vi "Set Digital State.vi"(8 "error in (no error)":errorcluster, 9 "Digital Control State (1: High)":i32(ring)=1 items=["Low", "High"], 10 "Line Number (1: line1)":i32(ring)=1 items=["line1"=1, "line2"=2, "line3"=3, "line4"=4, "line5"=5, "line6"=6], 11 "VISA resource name":refnum<visa-resource-name>) -> (0 "error out":errorcluster, 3 "VISA resource name out":refnum<visa-resource-name>)   [LabVIEW 2023, in "Keithley DMM6500 DAQ6500 Series.lvlib"]
doc: "Sets a digital I/O line high or low when the line is set for digital control and returns the state on the digital I/O lines."
uses:
  <instrlib>/Keithley DMM6500 DAQ6500 Series/Keithley DMM6500 DAQ6500 Series.lvlib
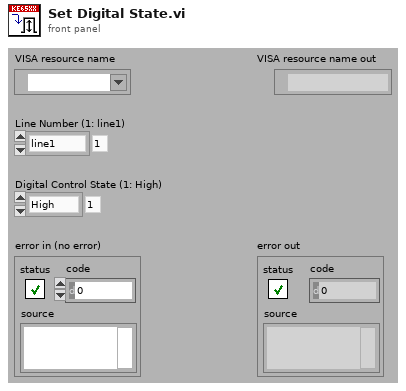
[diagram p1: front panel]
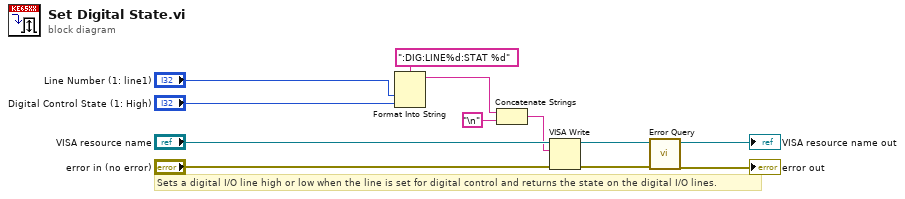
[diagram p0: block diagram]
diagram:
  # "Sets a digital I/O line high or low when the line is set for digital control and returns the state on the digital I/O lines."
  n1 = Format Into String(format string=":DIG:LINE%d:STAT %d", "Line Number (1: line1)", "Digital Control State (1: High)") -> (resulting string=w3:string)  [unwired: 2 in, 1 out]
  n2 = Concatenate Strings(w3, "\n") -> (w4:string)
  n3 = VISA Write(VISA resource name="VISA resource name", write buffer=w4, error in (no error)="error in (no error)") -> (VISA resource name out=w8:refnum<visa-resource-name>, error out=w7:errorcluster)  [unwired: 1 out]
  n4 = call <instrlib>:"Error Query.vi"("error in (no error)"=w7, "VISA resource name"=w8) -> ("error out"=→"error out":errorcluster, "VISA resource name out"=→"VISA resource name out":refnum<visa-resource-name>)  [unwired: 6 in, 2 out]
